vi "Read Log Text.vi"(11 "Jenkins Builder in":refnum<class "Jenkins Builder.lvclass">) -> (2 "Log Text":string, 3 "Jenkins Builder out":refnum<class "Jenkins Builder.lvclass">)   [LabVIEW 2014, in "Jenkins Builder.lvclass"]
uses:
  Jenkins Builder.lvclass
  Jenkins Builder.lvclass/Jenkins Builder.ctl
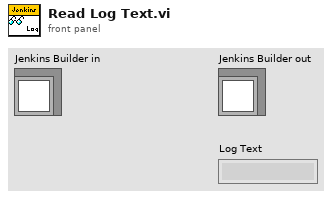
[diagram p1: front panel]
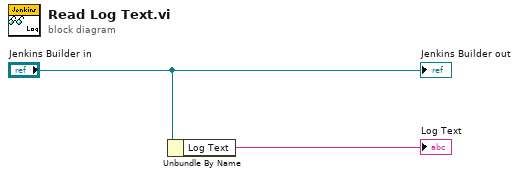
[diagram p0: block diagram]
diagram:
  n1 = Unbundle By Name("Jenkins Builder in") -> ("Log Text"=→"Log Text":string)
  "Jenkins Builder out" <- "Jenkins Builder in"
